vi "OnError.vi"(8 "Error In":errorcluster, 11 "JSON Tree In":variant) -> (0 "Error Out":errorcluster, 2 "Message":string, 3 "JSON Tree Out":variant)   [LabVIEW 2017, in "LiteAgentSDK.lvlib"]
uses:
  LiteAgentSDK.lvlib
  <vilib>/LVH/i3 JSON/JSON Parsing/Get Object Parameter Files/Get Object Parameter - String.vi
  <vilib>/LVH/i3 JSON/i3-json.lvlib
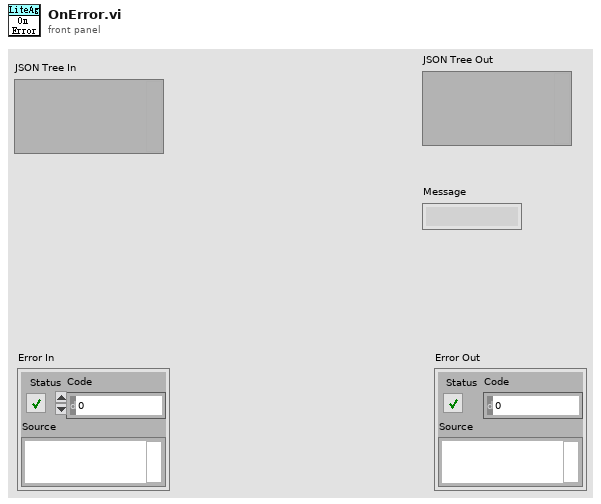
[diagram p1: front panel]
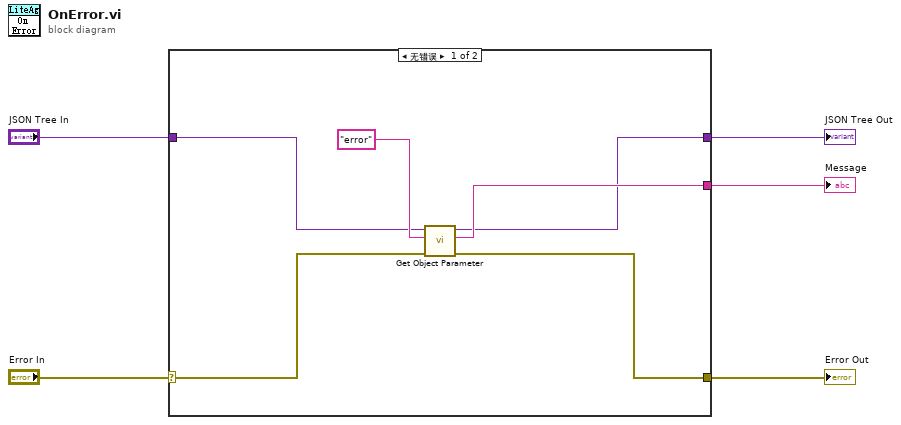
[diagram p0: block diagram]
diagram:
  n1 = case shown="无错误" "Error In" {
    selector: "Error In" -> [w8 w12]
    tunnel: [w7 w12] -> w4
    tunnel: "JSON Tree In" -> [w9 _]
    tunnel: [w10 _] -> w1
    tunnel: [w6 _] -> w2
    frame No Error {
      n2 = call-poly <vilib>:"Get Object Parameter.vi"("error in (no error)"=w8, "Parameter Name"="error", "JSON Tree In (JSON Object)"=w9) -> ("error out"=w7:errorcluster, "String Value"=w10:string, "JSON Tree Out Passthrough"=w6:variant)  [unwired: 5 in, 1 out]
    }
    frame Error {
    }
  }
  "Error Out" <- w4
  "JSON Tree Out" <- w2
  "Message" <- w1
